vi "Init.vi"(8 "error in (no error)":errorcluster) -> (0 "error out":errorcluster, 3 "Controller out":refnum<class "Controller.lvclass">)   [LabVIEW 2024, in "GUI.lvlib" / "Controller.lvclass"]
uses:
  Controller.lvclass
  Controller.lvclass/Controller.ctl
  <vilib>/drjdpowell/SQLite Library/SQL Connection/Open (path).vi
  <vilib>/drjdpowell/SQLite Library/SQL Connection/Open (string).vi
  <vilib>/AdvancedString/Path To Command Line String.vi
  <vilib>/drjdpowell/SQLite Library/SQL Connection/Connection.lvclass
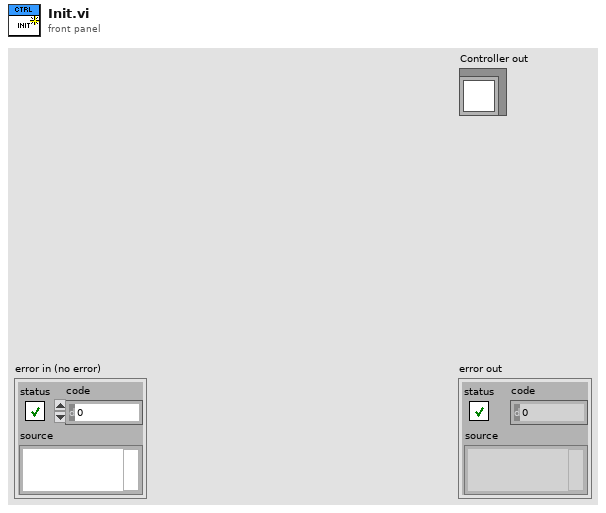
[diagram p1: front panel]
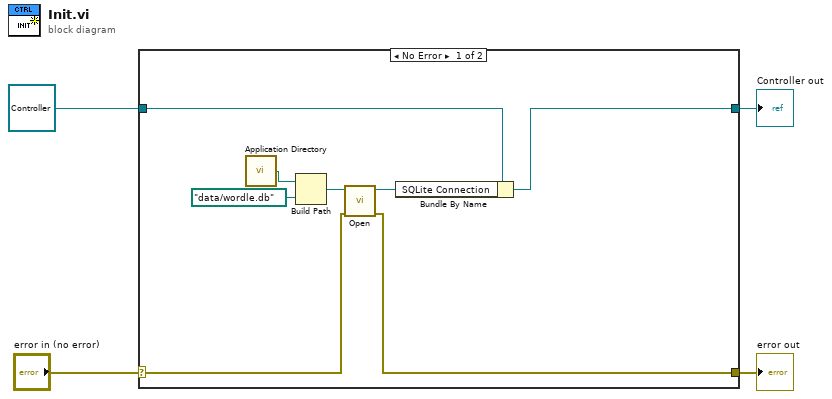
[diagram p0: block diagram]
diagram:
  n1 = case shown="No Error" "error in (no error)" {
    selector: "error in (no error)" -> [w5 w14]
    tunnel: [w6 w14] -> w3
    tunnel: [w7 w13] -> w1
    tunnel: refnum<class "Controller.lvclass"> refnum ("Controller in") -> [w8 w13]
    frame No Error {
      n2 = call <vilib>:"Application Directory.vi"() -> ("Application Directory"=w12:path)
      n3 = Build Path(base path=w12, name or relative path=path "data/wordle.db") -> (appended path=w10:path)
      n4 = call-poly <vilib>:"Open.vi"("error in (no error)"=w5, "db file"=w10) -> ("error out"=w6:errorcluster, "SQLite Connection"=w9:refnum<class "Connection.lvclass">)  [unwired: 8 in]
      n5 = Bundle By Name(cluster=w8, "SQLite Connection"=w9) -> (w7:refnum<class "Controller.lvclass">)
    }
    frame Error {
    }
  }
  "error out" <- w3
  "Controller out" <- w1
